vi "Channels.FilterByIDAndGlobal.vi"(10 "Station.ID":string, 11 "Channel":string) -> (3 "Use?":bool)   [LabVIEW 2015, in "Single Station Execution.lvlib"]
uses:
  Single Station Execution.lvlib
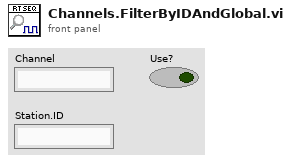
[diagram p1: front panel]
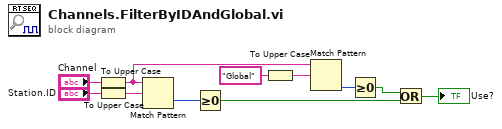
[diagram p0: block diagram]
diagram:
  n1 = To Upper Case(1:"Channel") -> (0:w3:string)
  n2 = To Upper Case(1:"Station.ID") -> (0:w2:string)
  n3 = Match Pattern(string=w3, regular expression=w2) -> (offset past match=w4:i32)  [unwired: 1 in, 3 out]
  n4 = Greater Or Equal To 0?(x=w4) -> (x >= 0?=w8:bool)
  n5 = To Upper Case(1:"Global" ("string")) -> (0:w1:string)
  n6 = Match Pattern(string=w3, regular expression=w1) -> (offset past match=w6:i32)  [unwired: 1 in, 3 out]
  n7 = Greater Or Equal To 0?(x=w6) -> (x >= 0?=w7:bool)
  n8 = Or(x=w7, y=w8) -> (x .or. y?=→"Use?":bool)
